vi "log-all-data.vi"(0 "log-file-byte-stream":refnum<file>, 1 "CSV Data Headings":string, 2 "adam5000:all-data-in":T3, 3 "log-start-time(mS)":u32, 4 "file open?":bool, 5 "error in (no error)":errorcluster, 6 "Log Filepath Selection":T2, 7 "Start Logging":bool, 8 "Enable Log Trigger":bool) -> (10 "appended path for log file":path, 11 "log-elapsed time":dbl format="%.2f", 12 "log-filepath-enable-state":T1(ring), 13 "Start Logging":bool, 14 "log-file-bytestream":refnum<file>, 15 "Logged Data String":string, 17 "log-start-time(mS)":u32, 18 "file open?":bool, 19 "error out":errorcluster)   [LabVIEW 2020]
uses:
  <vilib>/Utility/error.llb/DialogType.ctl
  controls/thermocouple-input-cluster.ctl
  controls/analog-input-cluster.ctl
  controls/analog-output-cluster.ctl
  controls/digitial-input-cluster.ctl
  controls/digital-output-cluster.ctl
  controls/adam-5000-all-module-datas.ctl
  controls/adam-5000-all-chassis-data.ctl
  csv-file-logging/filepath-selection.ctl
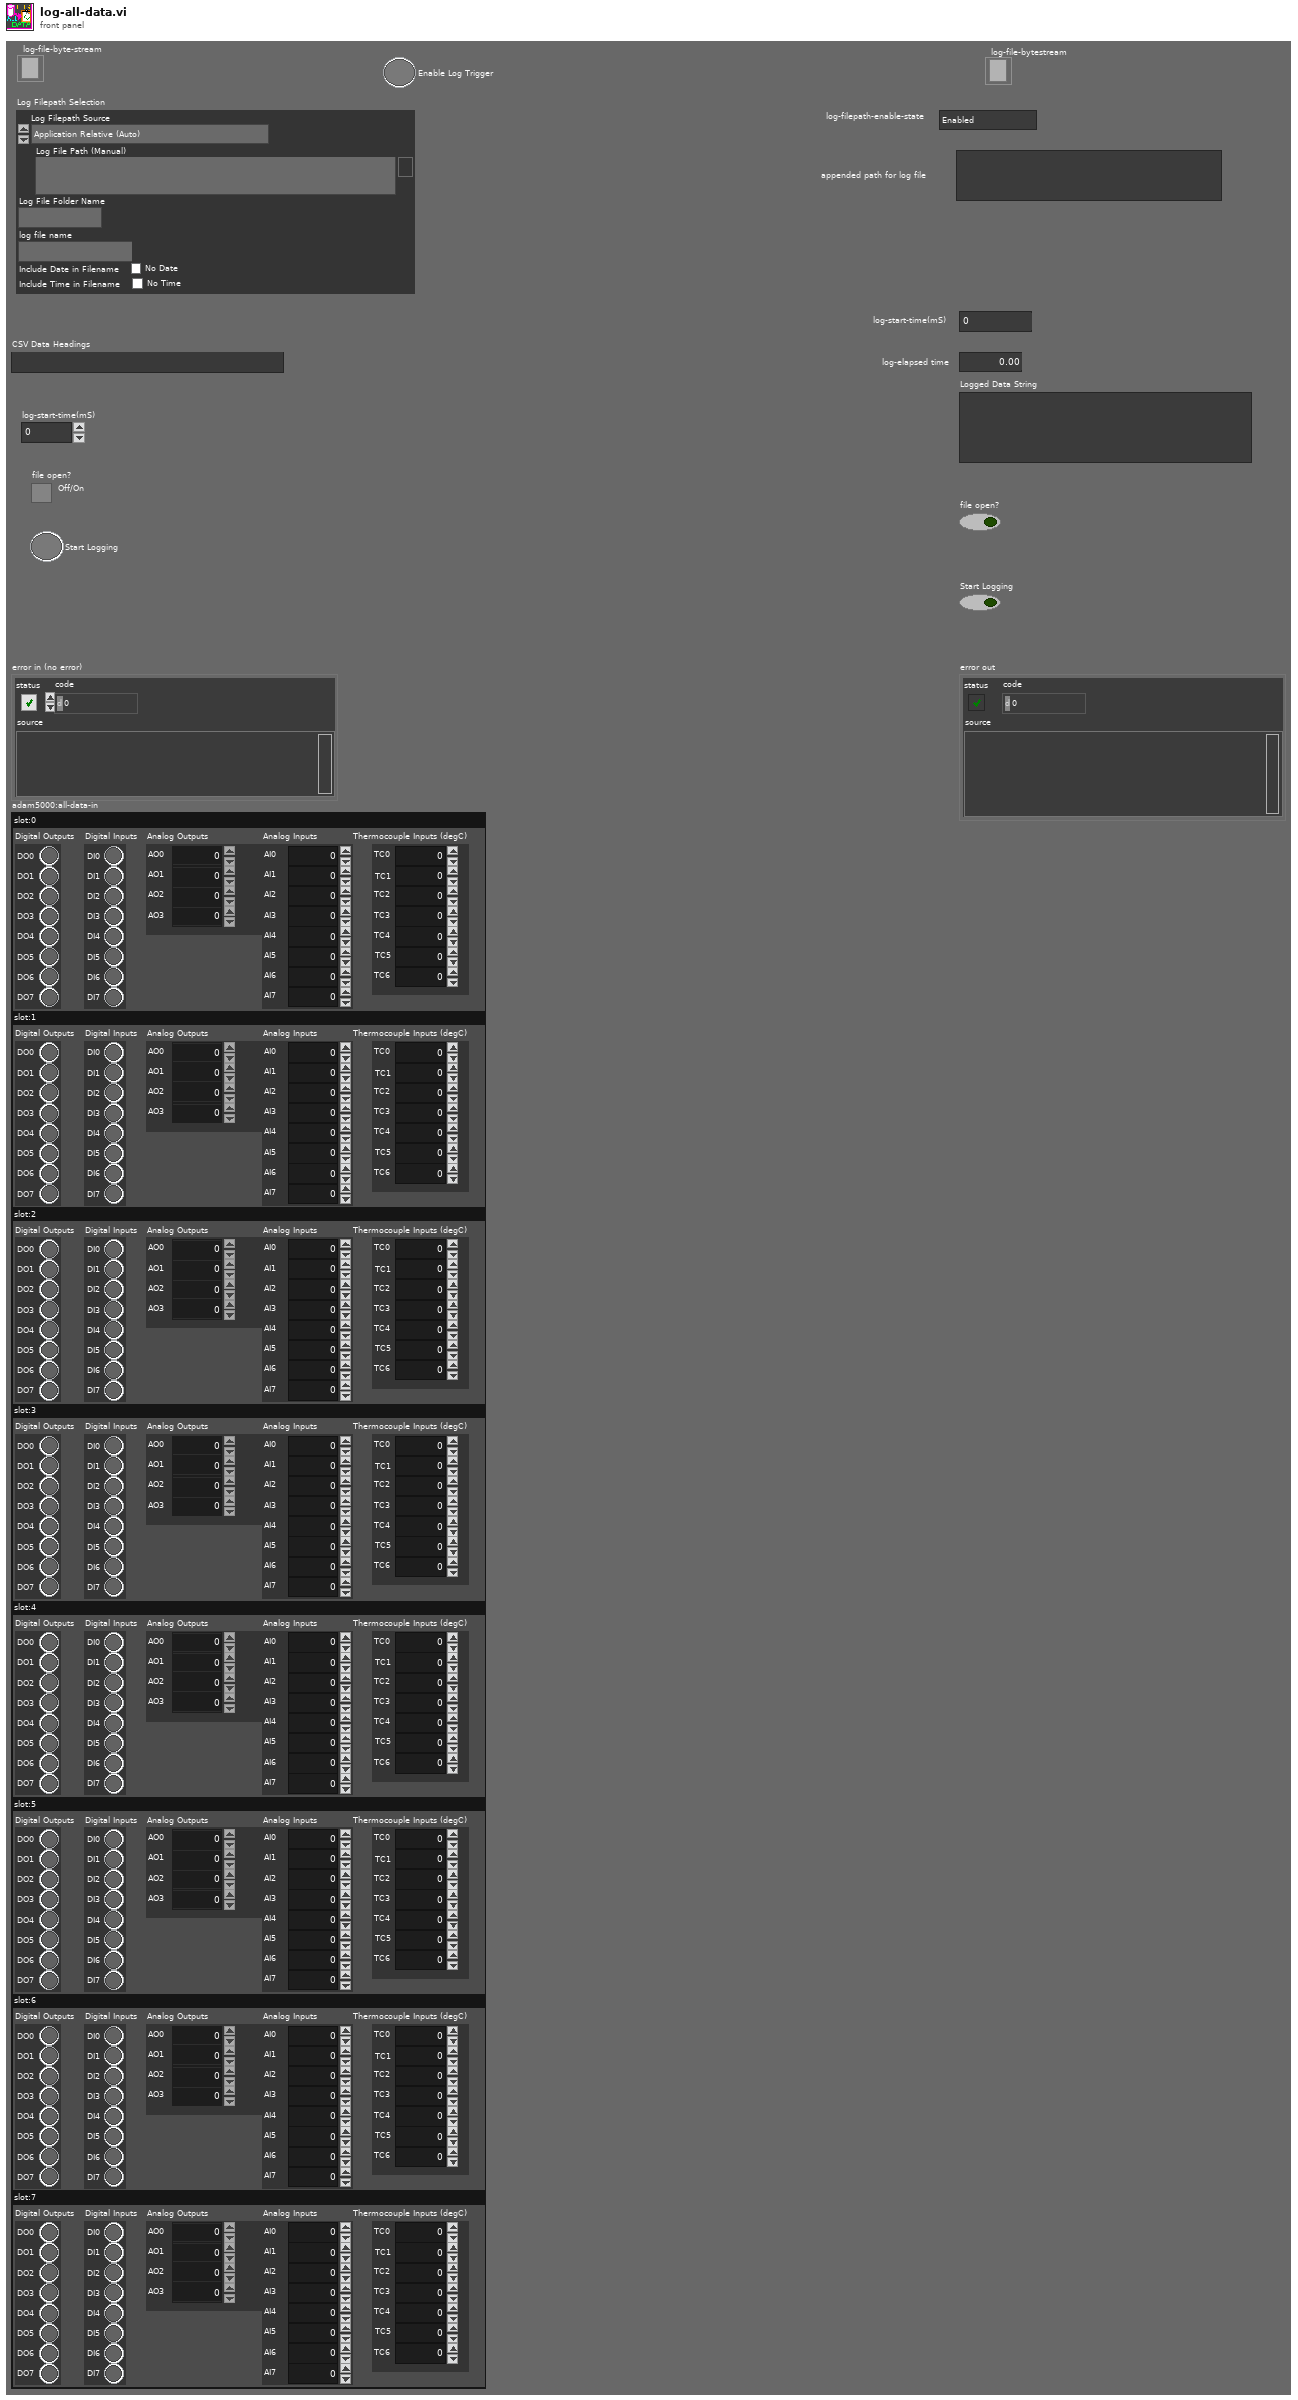
[diagram p1: front panel]
types:
  T1 = enum8{"Enabled", "Disabled", "Disabled and Grayed Out"}
  T2 = typedef "filepath-selection.ctl" = cluster{"Log Filepath Source":enum16{"Application Relative (Auto)", "VI Relative (Auto)", "Complete Path (Manual)"}, "Log File Path (Manual)":path, "Log File Folder Name":string, "log file name":string, "Include Date in Filename":bool, "Include Time in Filename":bool}
  T3 = typedef "adam-5000-all-chassis-data.ctl" = cluster{"slot:0":T4, "slot:1":T4, "slot:2":T4, "slot:3":T4, "slot:4":T4, "slot:5":T4, "slot:6":T4, "slot:7":T4}
  T4 = typedef "adam-5000-all-module-datas.ctl" = cluster{"Digital Outputs":T5, "Digital Inputs":T6, "Analog Outputs":T7, "Analog Inputs":T8, "Thermocouple Inputs (degC)":T9}
  T5 = typedef "digital-output-cluster.ctl" = cluster{"DO0":bool, "DO1":bool, "DO2":bool, "DO3":bool, "DO4":bool, "DO5":bool, "DO6":bool, "DO7":bool}
  T6 = typedef "digitial-input-cluster.ctl" = cluster{"DI0":bool, "DI1":bool, "DI2":bool, "DI3":bool, "DI4":bool, "DI5":bool, "DI6":bool, "DI7":bool}
  T7 = typedef "analog-output-cluster.ctl" = cluster{"AO0":dbl, "AO1":dbl, "AO2":dbl, "AO3":dbl}
  T8 = typedef "analog-input-cluster.ctl" = cluster{"AI0":dbl, "AI1":dbl, "AI2":dbl, "AI3":dbl, "AI4":dbl, "AI5":dbl, "AI6":dbl, "AI7":dbl}
  T9 = typedef "thermocouple-input-cluster.ctl" = cluster{"TC0":dbl, "TC1":dbl, "TC2":dbl, "TC3":dbl, "TC4":dbl, "TC5":dbl, "TC6":dbl}
  T10 = enum16{"open", "replace", "create", "open or create", "replace or create", "replace or create with confirmation"}
  T11 = typedef "DialogType.ctl" = u16
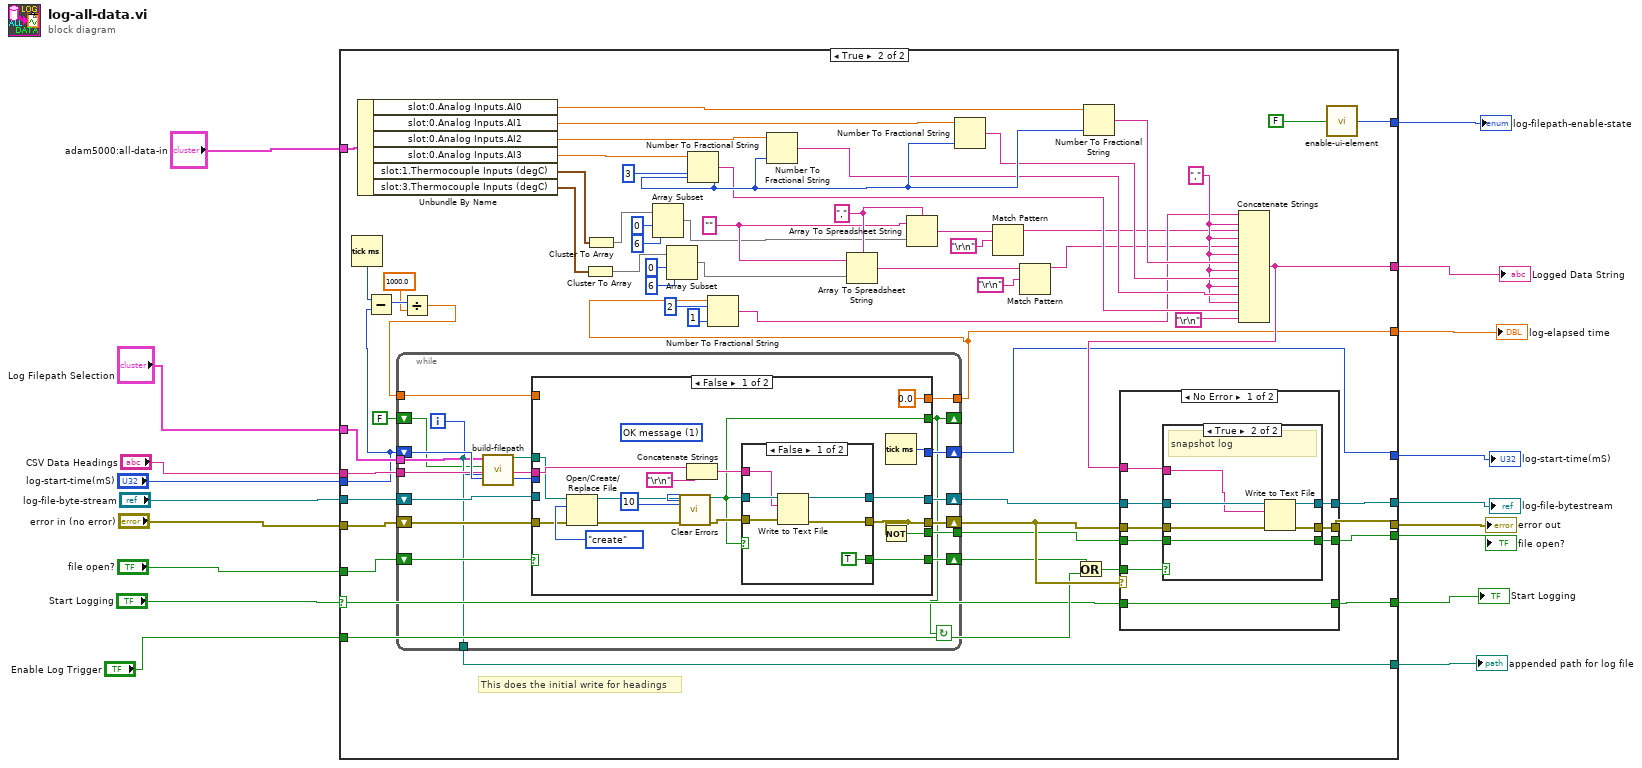
[diagram p0: block diagram]
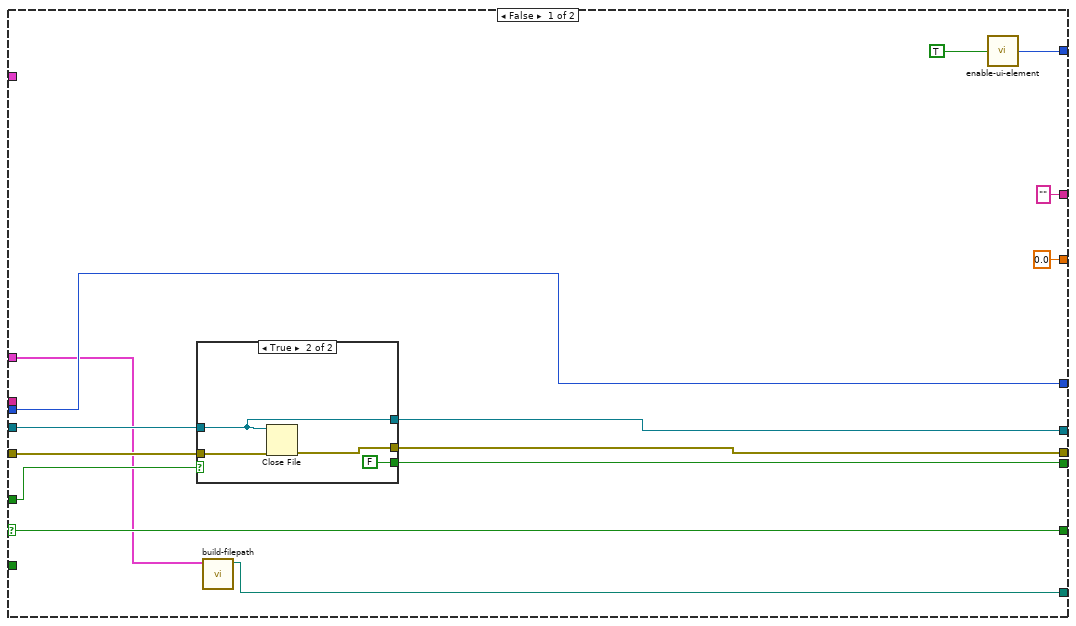
[diagram p2: hidden frame]
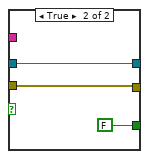
[diagram p4: hidden frame]
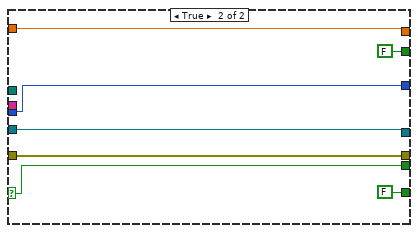
[diagram p5: hidden frame]
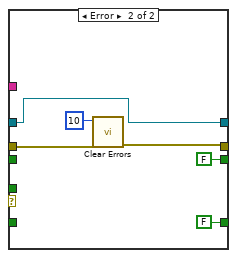
[diagram p7: hidden frame]
diagram:
  n1 = case shown="True" "Start Logging" {
    selector: "Start Logging" -> [w32 w48]
    tunnel: [w32 w47] -> w9
    tunnel: [w23 w98] -> w10
    tunnel: "adam5000:all-data-in" -> [_ w100]
    tunnel: [w30 w52] -> w12
    tunnel: "file open?" -> [w31 w97]
    tunnel: "error in (no error)" -> [w28 w96]
    tunnel: [w27 w89] -> w14
    tunnel: [w26 w90] -> w15
    tunnel: "log-file-byte-stream" -> [w29 w95]
    tunnel: [w25 w42] -> w17
    tunnel: "log-start-time(mS)" -> [w25 w43]
    tunnel: "CSV Data Headings" -> [_ w92]
    tunnel: ["" w54] -> w5
    tunnel: [0.0 w40] -> w4
    tunnel: [w19 w45] -> w3
    tunnel: "Enable Log Trigger" -> [_ w50]
    tunnel: "Log Filepath Selection" -> [w20 w46]
    frame False {
      n2 = case shown="True" w31 {
        selector: w31 -> [w33 _]
        tunnel: [w33 FALSE] -> w30
        tunnel: w29 -> [w35 w36]
        tunnel: w28 -> [w34 w38]
        tunnel: [w34 w37] -> w27
        tunnel: [w35 w36] -> w26
        frame False {
        }
        frame True {
          n3 = Close File(refnum=w36, error in=w38) -> (error out=w37:errorcluster)  [unwired: 1 out]
        }
      }
      n4 = call "build-filepath.vi"("Log Filepath Selection"=w20) -> ("appended path for log file"=w19:path)  [unwired: 9 in, 1 out]
      n5 = call "enable-ui-element.vi"("Enable UI Element"=TRUE) -> ("UI Element State"=w23:T1)  [unwired: 8 in]
    }
    frame True {
      w71 = "" ("format string")
      w78 = "," ("delimiter (Tab)")
      w73 = "," ("string")
      w80 = i16 3 ("precision (6)")
      # "This does the initial write for headings"
      n6 = Tick Count (ms)() -> (millisecond timer value=w94:u32)
      n7 = Unbundle By Name(w100) -> ("slot:0.Analog Inputs.AI0"=w88:dbl, "slot:0.Analog Inputs.AI1"=w85:dbl, "slot:0.Analog Inputs.AI2"=w84:dbl, "slot:0.Analog Inputs.AI3"=w87:dbl, "slot:1.Thermocouple Inputs (degC)"=w82:T9, "slot:3.Thermocouple Inputs (degC)"=w81:T9)
      n8 = Subtract(x=w94, y=w43) -> (x-y=w93:u32)
      n9 = Divide(x=w93, y=1000.0) -> (x/y=w41:dbl)
      n10 = while {
        tunnel: w92 -> [w112]
        tunnel: [w109] -> w53
        tunnel: w46 -> [w107]
        tunnel: [w106] -> w45
        shift-right: [w108] -> w49
        shift-left: w97 -> [w117]
        shift-right: [w110] -> w55
        shift-left: w96 -> [w116]
        shift-right: [w111] -> w91
        shift-left: w95 -> [w115]
        shift-right: [w114] -> w42
        shift-left: w43 -> [w113]
        shift-right: [w103] -> _
        shift-left: FALSE ("specific error cleared?") -> [w104]
        tunnel: w41 -> [w101]
        tunnel: [w102] -> w40
        i -> [w105]
        stop <- w103 continue-if-true
        n11 = call "build-filepath.vi"("increment file-number"=w105, "increment filename?"=w104, "Log Filepath Selection"=w107) -> ("appended path for log file"=w106:path)  [unwired: 7 in, 1 out]
        n12 = case shown="False" w117 {
          selector: w117 -> [_ w150]
          tunnel: w116 -> [w133 w149]
          tunnel: [w123 w149] -> w110
          tunnel: [w132 w150] -> w109
          tunnel: [w124 w147] -> w111
          tunnel: w115 -> [_ w147]
          tunnel: [w131 w148] -> w114
          tunnel: w113 -> [_ w148]
          tunnel: w112 -> [w129 _]
          tunnel: [w119 FALSE ("x")] -> w108
          tunnel: w106 -> [w122 _]
          tunnel: [w120 FALSE ("specific error cleared?")] -> w103
          tunnel: [0.0 w144] -> w102
          tunnel: w101 -> [_ w144]
          frame False {
            (unwired) T11 1 items=["no dialog", "OK message", "continue or stop message", "OK message + warnings", "continue/stop + warnings"] ("type of dialog (OK msg:1)")
            n13 = Open/Create/Replace File(file path (use dialog)=w122, error in=w133, operation (0:open)=T10."create") -> (refnum out=w126:refnum<file>, error out=w128:errorcluster)  [unwired: 3 in, 1 out]
            n14 = call <vilib>:"Clear Errors.vi"("error in (no error)"=w128, "specific error code to clear (0: all)"=10 ("error code (no error:0)")) -> ("error out"=w125:errorcluster, "specific error cleared?"=w120:bool)  [unwired: 4 in]
            n15 = Concatenate Strings(w129, "\r\n") -> (w121:string)
            n16 = case shown="False" w120 {
              tunnel: w126 -> [w140 w143]
              tunnel: w125 -> [w139 w142]
              tunnel: [w138 w143] -> w124
              tunnel: [w137 w142] -> w123
              tunnel: w121 -> [w136 _]
              tunnel: [TRUE ("x") FALSE ("x")] -> w119
              frame False {
                n17 = Write to Text File(file (use dialog)=w140, text=w136, error in=w139) -> (refnum out=w138:refnum<file>, error out=w137:errorcluster)  [unwired: 1 in, 1 out]
              }
              frame True {
              }
            }
            n18 = Not(x=w123) -> (.not. x?=w132:bool)
            n19 = Tick Count (ms)() -> (millisecond timer value=w131:u32)
          }
          frame True {
          }
        }
      }
      n20 = Cluster To Array(cluster=w81) -> (array=w58:dbl[])
      n21 = Cluster To Array(cluster=w82) -> (array=w64:dbl[])
      n22 = Array Subset(array=w64, index=0, length=6) -> (w61:dbl[])
      n23 = Array Subset(array=w58, index=0, length=6) -> (w57:dbl[])
      n24 = Number To Fractional String(number=w87, precision (6)=w80) -> (F-format string=w77:string)  [unwired: 2 in]
      n25 = Number To Fractional String(number=w40, width (-)=i16 2, precision (6)=i16 1) -> (F-format string=w72:string)  [unwired: 1 in]
      n26 = Number To Fractional String(number=w84, precision (6)=w80) -> (F-format string=w76:string)  [unwired: 2 in]
      n27 = Array To Spreadsheet String(delimiter (Tab)=w78, array=w57, 3:w71) -> (spreadsheet string=w67:string)
      n28 = Array To Spreadsheet String(delimiter (Tab)=w78, array=w61, 3:w71) -> (spreadsheet string=w70:string)
      n29 = Number To Fractional String(number=w85, precision (6)=w80) -> (F-format string=w75:string)  [unwired: 2 in]
      n30 = Match Pattern(string=w70, regular expression="\r\n") -> (before substring=w69:string)  [unwired: 1 in, 3 out]
      n31 = Match Pattern(string=w67, regular expression="\r\n") -> (before substring=w65:string)  [unwired: 1 in, 3 out]
      n32 = Or(x=w49, y=w50) -> (x .or. y?=w51:bool)
      n33 = Number To Fractional String(number=w88, precision (6)=w80) -> (F-format string=w74:string)  [unwired: 2 in]
      n34 = Concatenate Strings(w72, w73, w69, w73, w65, w73, w74, w73, w75, w73, w76, w73, w77, "\r\n") -> (w54:string)
      n35 = case shown="No Error" w55 {
        tunnel: w91 -> [w159 w172]
        tunnel: [w158 w172] -> w90
        tunnel: w55 -> [w157 w173]
        tunnel: [w156 w171] -> w89
        tunnel: w54 -> [w155 _]
        tunnel: w51 -> [w154 _]
        tunnel: w53 -> [w152 _]
        tunnel: [w153 FALSE] -> w52
        tunnel: w48 -> [w151 _]
        tunnel: [w151 FALSE] -> w47
        frame No Error {
          n36 = case shown="True" w154 {
            tunnel: w159 -> [w162 w168]
            tunnel: [w162 w167] -> w158
            tunnel: w157 -> [w161 w166]
            tunnel: [w161 w165] -> w156
            tunnel: w155 -> [_ w164]
            tunnel: [w160 w163] -> w153
            tunnel: w152 -> [w160 w163]
            frame False {
            }
            frame True {
              # "snapshot log"
              n37 = Write to Text File(file (use dialog)=w168, text=w164, error in=w166) -> (refnum out=w167:refnum<file>, error out=w165:errorcluster)  [unwired: 1 in, 1 out]
            }
          }
        }
        frame Error {
          n38 = call <vilib>:"Clear Errors.vi"("error in (no error)"=w173, "specific error code to clear (0: all)"=10) -> ("error out"=w171:errorcluster)  [unwired: 4 in, 1 out]
        }
      }
      n39 = call "enable-ui-element.vi"("Enable UI Element"=FALSE) -> ("UI Element State"=w98:T1)  [unwired: 8 in]
    }
  }
  "log-start-time(mS)" <- w17
  "log-file-bytestream" <- w15
  "error out" <- w14
  "file open?" <- w12
  "appended path for log file" <- w3
  "log-filepath-enable-state" <- w10
  "Start Logging" <- w9
  "Logged Data String" <- w5
  "log-elapsed time" <- w4
